vi "Parse Scripts.vi"   [LabVIEW 2017]
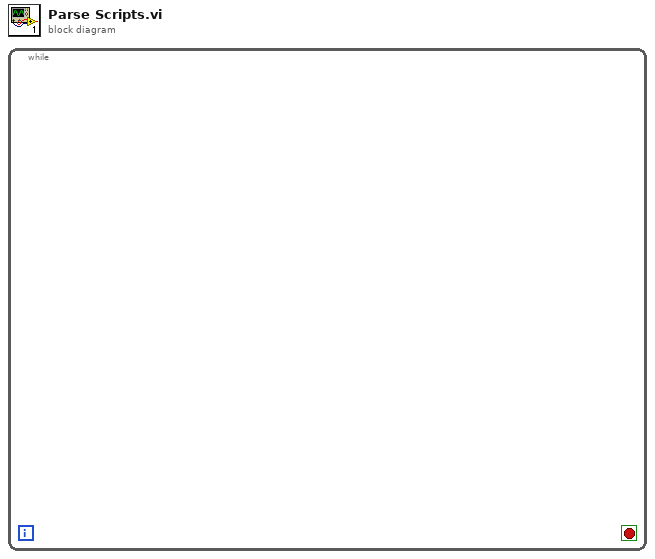
[diagram p0: block diagram]
diagram:
  n1 = while {
    stop <- _ stop-if-true
  }
